vi "Demo1_Requestor.vi"() -> ()   [LabVIEW 2019]
uses:
  response -- cluster.ctl
  <vilib>/LabVIEW Open Source Project/OpenSerializer JKI JSON/Serializer.JSON.lvclass
  C:/Program Files (x86)/National Instruments/LabVIEW 2019/vi.lib/LabVIEW Open Source Project/OpenSerializer/Serializer/Serializer.lvclass
  <vilib>/LabVIEW Open Source Project/MQTT Connection/MQTT_Base/Base Class/MQTT_Base.lvclass/MQTT_Base.ctl
  <vilib>/LabVIEW Open Source Project/MQTT Client/Client class/Client.lvclass/Client.ctl
  <vilib>/LabVIEW Open Source Project/MQTT Control Packets/Control Packets/ControlPacket/ControlPacket.lvclass/ControlPacket.ctl
  request -- cluster.ctl
  <vilib>/LabVIEW Open Source Project/MQTT TCP Connection/MQTT_TCP/Connection/TCPConnection.lvclass
  C:/Program Files (x86)/National Instruments/LabVIEW 2019/vi.lib/LabVIEW Open Source Project/MQTT Connection/MQTT_Connection/Connection/Connection.lvclass
  <vilib>/LabVIEW Open Source Project/MQTT Client/Client class/Client.lvclass
  C:/Program Files (x86)/National Instruments/LabVIEW 2019/vi.lib/LabVIEW Open Source Project/MQTT Connection/MQTT_Base/Base Class/MQTT_Base.lvclass
  <vilib>/LabVIEW Open Source Project/OpenSerializer/Serializer.FlattenedString/Serializer.FlattenedString.lvclass
  <vilib>/LabVIEW Open Source Project/MQTT Control Packets/Control Packets/PUBLISH/PUBLISH.lvclass
  C:/Program Files (x86)/National Instruments/LabVIEW 2019/vi.lib/LabVIEW Open Source Project/MQTT Control Packets/Control Packets/ControlPacket/ControlPacket.lvclass
  <vilib>/LabVIEW Open Source Project/OpenSerializer/Serializer/Serializer.lvclass
  <vilib>/LabVIEW Open Source Project/MQTT Connection/MQTT_Base/Base Class/MQTT_Base.lvclass
  <vilib>/LabVIEW Open Source Project/OpenSerializer.Base64/Serializer.Base64.lvclass
  <vilib>/LabVIEW Open Source Project/MQTT Control Packets/Control Packets/ControlPacket/ControlPacket.lvclass
panel:
  out "state":dbl
  out "response topic":string="getState"
  out "response":T1
  in  "response tag":string="getState"
  in  "Send Request":bool
  in  "payload":string
  in  "request":string="getState"
  out "last error":errorcluster
  in  "Connection":bool
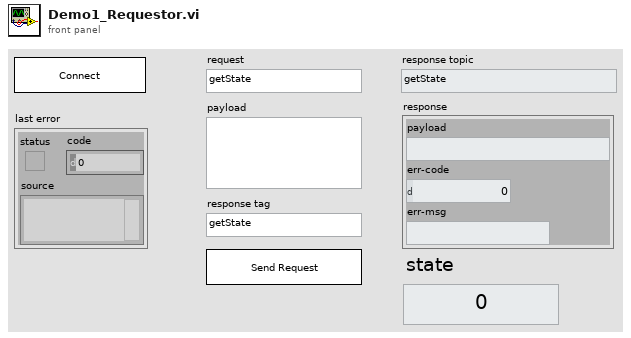
[diagram p1: front panel]
types:
  T1 = typedef "response -- cluster.ctl" = cluster{"payload":string, "err-code":i32, "err-msg":string}
  T2 = cluster{"remoteName":string, "state":dbl, "selfName":string}
  T3 = typedef "MQTT Client.lvlib/Client.lvclass/Public Events -- cluster.ctl" = cluster{"Connection Status":refnum<user-event>, "Connected":refnum<user-event>, "Application Message":refnum<user-event>}
  T4 = typedef "MQTT Base.lvlib/MQTT_Base.lvclass/Public Events -- cluster.ctl" = cluster{"Stop Event":refnum<user-event>, "Error Event":refnum<user-event>, "Inbound Message":refnum<user-event>}
  T5 = typedef "request -- cluster.ctl" = cluster{"payload":string, "responseURI":string}
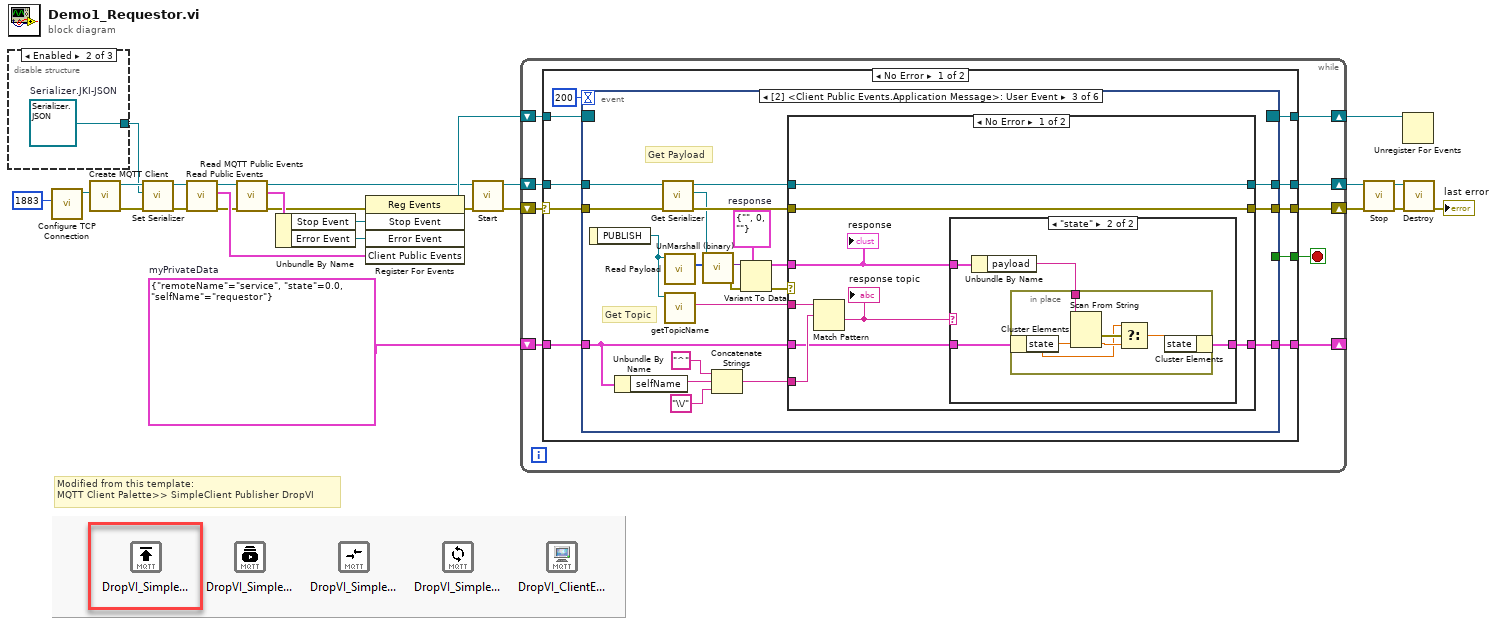
[diagram p0: block diagram]
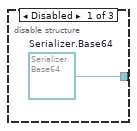
[diagram p2: hidden frame]
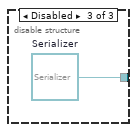
[diagram p3: hidden frame]
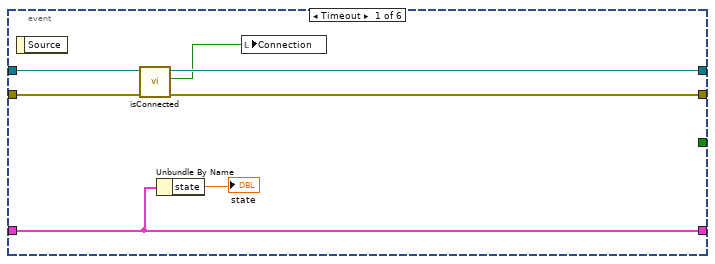
[diagram p4: hidden frame]
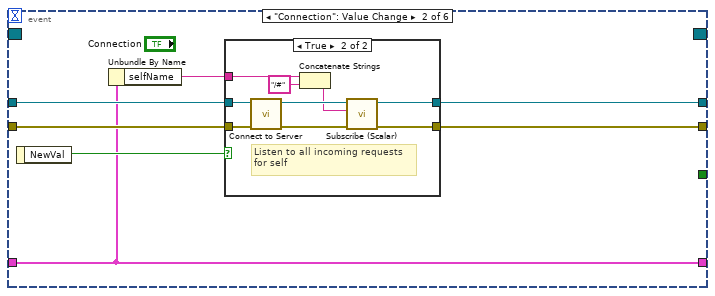
[diagram p5: hidden frame]
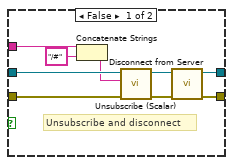
[diagram p6: hidden frame]
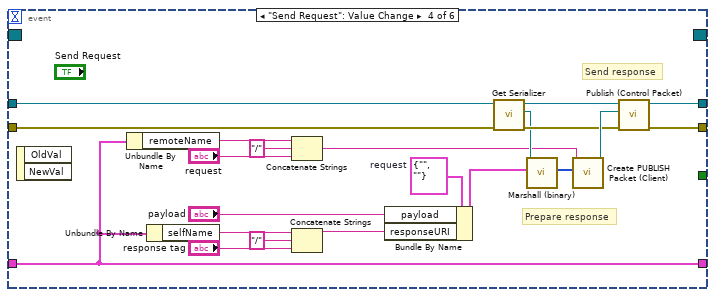
[diagram p9: hidden frame]
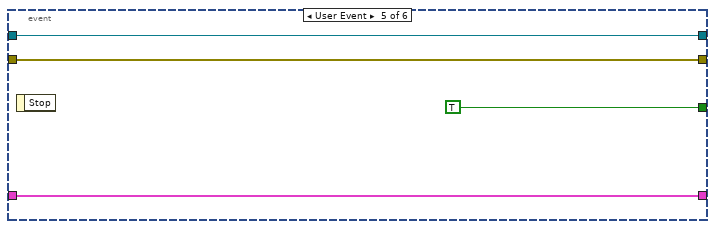
[diagram p10: hidden frame]
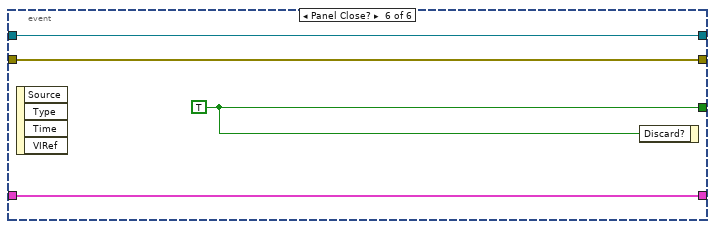
[diagram p11: hidden frame]
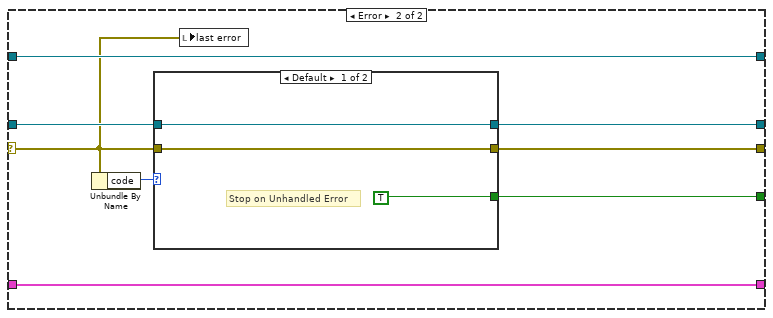
[diagram p12: hidden frame]
diagram:
  w1 = T2 {"remoteName"="service", "state"=0.0, "selfName"="requestor"}  # myPrivateData
  # "Modified from this template:\nMQTT Client Palette>> SimpleClient Publisher DropVI"
  n1 = disable-structure shown="Enabled" {
    disable-tunnel: [w27 w28 w29] -> w2
    frame Disabled {
      w27 = refnum<class "Serializer.Base64.lvclass"> refnum  # Serializer.Base64
    }
    frame Enabled {
      w28 = refnum<class "Serializer.JSON.lvclass"> refnum  # Serializer.JKI-JSON
    }
    frame Disabled {
      w29 = refnum<class "Serializer.lvclass"> refnum  # Serializer
    }
  }
  n2 = call <vilib>:"Configure TCP Connection.vi"("remote port (80)"=u16 1883) -> ("TCPConnection"=w7:refnum<class "TCPConnection.lvclass">)  [unwired: 9 in, 1 out]
  n3 = call <vilib>:"Create MQTT Client.vi"("Connection Configuration"=w7) -> ("error out"=w4:errorcluster, "Client out"=w6:refnum<class "Client.lvclass">)  [unwired: 9 in]
  n4 = call <vilib>:"Set Serializer.vi"("error in (no error)"=w4, "Serializer (default: Flattened String)"=w2, "MQTT_Base"=w6) -> ("error out"=w3:errorcluster, "MQTT_Base out"=w5:refnum<class "Client.lvclass">)  [unwired: 7 in]
  n5 = call <vilib>:"Read Public Events.vi"("error in (no error)"=w3, "Client in"=w5) -> ("error out"=w10:errorcluster, "Client Public Events"=w12:T3, "Client out"=w9:refnum<class "Client.lvclass">)  [unwired: 7 in]
  n6 = call <vilib>:"Read MQTT Public Events.vi"("error in (no error)"=w10, "MQTT_Base in"=w9) -> ("error out"=w11:errorcluster, "MQTT Public Events"=w19:T4, "MQTT_Base out"=w14:refnum<class "Client.lvclass">)  [unwired: 7 in]
  n7 = Unbundle By Name(w19) -> ("Stop Event"=w17:refnum<user-event>, "Error Event"=w18:refnum<user-event>)
  n8 = register-events(error in=w11, w17, w18, w12) -> (reference out=w15:refnum<event-registration>, error out=w13:errorcluster)  [unwired: 1 in]
  n9 = call <vilib>:"Start.vi"("error in (no error)"=w13, "MQTT_Base in"=w14) -> ("error out"=w25:errorcluster, "MQTT_Base out"=w24:refnum<class "Client.lvclass">)  [unwired: 7 in, 1 out]
  n10 = while {
    shift-right: [w37] -> w16
    shift-left: w15 -> [w38]
    shift-right: [w34] -> w21
    shift-left: w24 -> [w35]
    shift-right: [w36] -> w23
    shift-left: w25 -> [w32]
    shift-right: [w31] -> _
    shift-left: w1 -> [w30]
    stop <- w33 stop-if-true
    n11 = case shown="No Error" w32 {
      selector: w32 -> [w41 w153]
      tunnel: w38 -> [w48 w159]
      tunnel: [w47 w159] -> w37
      tunnel: [w46 w155] -> w36
      tunnel: w35 -> [w44 w157]
      tunnel: [w43 w156] -> w34
      tunnel: [w42 w154] -> w33
      tunnel: [w40 w152] -> w31
      tunnel: w30 -> [w39 w152]
      frame No Error {
        n12 = event shown="[2] <Client Public Events.Application Message>: User Event" {
          selector: w48 -> [_ _ _ _ _ _]
          dyn-events: [_ _ _ _ _ _] -> w47
          timeout: 200 -> [_ _ _ _ _ _]
          tunnel: w41 -> [w53 w58 w95 w133 w147 w149]
          tunnel: [w52 w59 w100 w142 w147 w149] -> w46
          tunnel: [_ _ _ _ TRUE w151] -> w42
          tunnel: w44 -> [w55 w62 w97 w141 w145 w150]
          tunnel: [w54 w60 w101 w143 w145 w150] -> w43
          tunnel: [w51 w57 w91 w123 w144 w148] -> w40
          tunnel: w39 -> [w51 w57 w87 w123 w144 w148]
          event Timeout {
            n13 = event-data() -> ()  [unwired: 1 in, 1 out]
            n14 = call <vilib>:"isConnected.vi"("error in (no error)"=w53, "Client in"=w55) -> ("error out"=w52:errorcluster, "connected"=w49:bool, "Client out"=w54:refnum<class "Client.lvclass">)  [unwired: 7 in]
            n15 = Unbundle By Name(w51) -> ("state"=→"state":dbl)
            n16 = local write "Connection"(w49) -> ()
          }
          event "Connection": Value Change {
            n17 = event-data() -> ("NewVal"=w61:bool)  [unwired: 1 in]
            n18 = Unbundle By Name(w57) -> ("selfName"=w56:string)
            n19 = case shown="True" w61 {
              tunnel: w62 -> [w66 w80]
              tunnel: [w71 w77] -> w60
              tunnel: [w70 w75] -> w59
              tunnel: w58 -> [w64 w79]
              tunnel: w56 -> [w68 w74]
              frame False {
                # "Unsubscribe and disconnect"
                n20 = Concatenate Strings(w68, "/#" ("string")) -> (w63:string)
                n21 = call <vilib>:"Unsubscribe (Scalar).vi"("error in (no error)"=w64, "Topic Filter"=w63, "Client in"=w66) -> ("error out"=w65:errorcluster, "Client out"=w67:refnum<class "Client.lvclass">)  [unwired: 6 in, 1 out]
                n22 = call <vilib>:"Disconnect from Server.vi"("error in (no error)"=w65, "Client in"=w67) -> ("error out"=w70:errorcluster, "Client out"=w71:refnum<class "Client.lvclass">)  [unwired: 7 in, 1 out]
              }
              frame True {
                # "Listen to all incoming requests\nfor self"
                n23 = call <vilib>:"Connect to Server.vi"("error in (no error)"=w79, "Client in"=w80) -> ("error out"=w76:errorcluster, "Client out"=w78:refnum<class "Client.lvclass">)  [unwired: 6 in, 2 out]
                n24 = Concatenate Strings(w74, "/#" ("string")) -> (w72:string)
                n25 = call <vilib>:"Subscribe (Scalar).vi"("error in (no error)"=w76, "Topic Filter"=w72, "Client in"=w78) -> ("error out"=w75:errorcluster, "Client out"=w77:refnum<class "Client.lvclass">)  [unwired: 6 in, 1 out]
              }
            }
          }
          event User Event {
            w84 = T1 {"payload"="", "err-code"=0, "err-msg"=""}  # response
            # "Get Payload"
            # "Get Topic"
            n26 = event-data() -> ("PUBLISH"=w99:refnum<class "PUBLISH.lvclass">)  [unwired: 1 in]
            n27 = Unbundle By Name(w87) -> ("selfName"=w88:string)
            n28 = call <vilib>:"Get Serializer.vi"("error in (no error)"=w95, "MQTT_Base"=w97) -> ("error out"=w96:errorcluster, "Serializer"=w92:refnum<class "Serializer.lvclass">, "MQTT_Base out"=w98:refnum<class "Client.lvclass">)  [unwired: 7 in]
            n29 = call <vilib>:"Read Payload.vi"("ControlPacket in"=w99) -> ("Payload"=w94:u8[])  [unwired: 9 in, 1 out]
            n30 = call <vilib>:"getTopicName.vi"("PUBLISH in"=w99) -> ("Topic"=w83:string)  [unwired: 8 in, 2 out]
            n31 = call <vilib>:"UnMarshall (binary).vi"("Bytes"=w94, "Serializer in"=w92) -> ("error out"=w81:errorcluster, "Variant"=w93:variant)  [unwired: 7 in, 1 out]
            n32 = Concatenate Strings("^" ("string"), w88, "\\/" ("string")) -> (w82:string)
            n33 = Variant To Data(error in=w81, type=w84, Variant=w93) -> (data=w85:T1, error out=w86:errorcluster)
            n34 = case shown="No Error" w86 {
              tunnel: [w108 w122] -> w101
              tunnel: [w107 w121] -> w100
              tunnel: w85 -> [w109 _]
              tunnel: w98 -> [w108 w122]
              tunnel: w96 -> [w107 w121]
              tunnel: [w103 w120] -> w91
              tunnel: w87 -> [w104 w120]
              tunnel: w83 -> [w106 _]
              tunnel: w82 -> [w105 _]
              frame No Error {
                n35 = Match Pattern(string=w106, regular expression=w105) -> (after substring=w102:string)  [unwired: 1 in, 3 out]
                "response topic" <- w102
                n36 = case shown="\"state\"" w102 {
                  tunnel: w109 -> [_ w114]
                  tunnel: w104 -> [w110 w113]
                  tunnel: [w110 w112] -> w103
                  frame Default {
                  }
                  frame "state" {
                    n37 = Unbundle By Name(w114) -> ("payload"=w111:string)
                    n38 = in-place {
                      in-place-border: w111 -> [w119]
                      n39 = in-place-cluster #1(w113) -> ("state"=w115:dbl)
                      n40 = Scan From String(input string=w119, default 1=w115) -> (error out=w118:errorcluster, output 1=w116:dbl)  [unwired: 3 in, 2 out]
                      n41 = Select(t=w115, s=w118, f=w116) -> (s? t:f=w117:dbl)
                      n42 = in-place-cluster #1("state"=w117) -> (w112:T2)
                    }
                  }
                }
                "response" <- w109
              }
              frame Error {
                # "Invalid Packet Format.\nReject response."
              }
            }
          }
          event "Send Request": Value Change {
            w134 = T5 {"payload"="", "responseURI"=""}  # request
            # "Prepare response"
            # "Send response"
            n43 = event-data() -> ()  [unwired: 1 in, 2 out]
            n44 = Unbundle By Name(w123) -> ("remoteName"=w130:string)
            n45 = Unbundle By Name(w123) -> ("selfName"=w128:string)
            n46 = Concatenate Strings(w130, "/", "request") -> (w129:string)
            n47 = Concatenate Strings(w128, "/", "response tag") -> (w124:string)
            n48 = Bundle By Name(cluster=w134, "payload"="payload", "responseURI"=w124) -> (w135:T5)
            n49 = call <vilib>:"Get Serializer.vi"("error in (no error)"=w133, "MQTT_Base"=w141) -> ("error out"=w138:errorcluster, "Serializer"=w136:refnum<class "Serializer.lvclass">, "MQTT_Base out"=w137:refnum<class "Client.lvclass">)  [unwired: 7 in]
            n50 = call <vilib>:"Marshall (binary).vi"("Variant"=w135, "Serializer in"=w136) -> ("Bytes"=w139:u8[])  [unwired: 7 in, 2 out]
            n51 = call <vilib>:"Create PUBLISH Packet (Client).vi"("Payload"=w139, "Topic Name"=w129) -> ("PUBLISH"=w140:refnum<class "PUBLISH.lvclass">)  [unwired: 6 in, 3 out]
            n52 = call <vilib>:"Publish (Control Packet).vi"("error in (no error)"=w138, "PUBLISH"=w140, "Client in"=w137) -> ("error out"=w142:errorcluster, "Client out"=w143:refnum<class "Client.lvclass">)  [unwired: 6 in, 1 out]
          }
          event User Event {
            n53 = event-data() -> ()  [unwired: 1 in, 1 out]
          }
          event Panel Close? {
            w151 = TRUE
            n54 = event-data() -> ()  [unwired: 1 in, 4 out]
            n55 = event-data("Discard?"=w151) -> ()  [unwired: 1 in, 1 out]
          }
        }
      }
      frame Error {
        n56 = Unbundle By Name(w153) -> ("code"=w158:i32)
        n57 = case shown="Default" w158 {
          tunnel: w157 -> [w162 w163]
          tunnel: [w162 w163] -> w156
          tunnel: w153 -> [w161 _]
          tunnel: [w161 _] -> w155
          tunnel: [TRUE _] -> w154
          frame Default {
            # "Stop on Unhandled Error"
          }
          frame 56, 63, 66 {
            # "Disconnected"
          }
        }
        n58 = local write "last error"(w153) -> ()
      }
    }
  }
  n59 = call <vilib>:"Stop.vi"("error in (no error)"=w23, "MQTT_Base in"=w21) -> ("error out"=w22:errorcluster, "MQTT_Base out"=w20:refnum<class "Client.lvclass">)  [unwired: 7 in, 1 out]
  n60 = Unregister For Events(event registration refnum=w16) -> ()  [unwired: 1 in, 1 out]
  n61 = call <vilib>:"Destroy.vi"("error in (no error)"=w22, "MQTT_Base in"=w20) -> ("error out"=→"last error":errorcluster)  [unwired: 8 in, 1 out]
